vi "Read Configuration Parameters.vi"(8 "error in (no error)":errorcluster, 10 "refnum":T1, 11 "Configuration in":refnum<class "Configuration.lvclass">) -> (0 "error out":errorcluster, 2 "refnum out":T1, 3 "Configuration out":refnum<class "Configuration.lvclass">)   [LabVIEW 2016, in "Configuration.lvlib" / "Configuration.lvclass"]
uses:
  <userlib>/Configuration Dialog Actor/Configuration.lvclass
  <vilib>/Utility/config.llb/Config Data RefNum.ctl
  <userlib>/Configuration Dialog Actor/Configuration.lvclass/Configuration.ctl
  <vilib>/Utility/config.llb/NI_LVConfig.lvlib
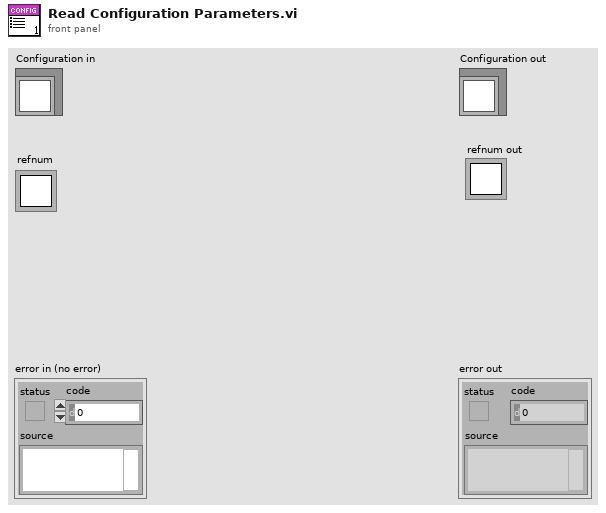
[diagram p1: front panel]
types:
  T1 = typedef "NI_LVConfig.lvlib/Config Data RefNum.ctl" = refnum<k1>
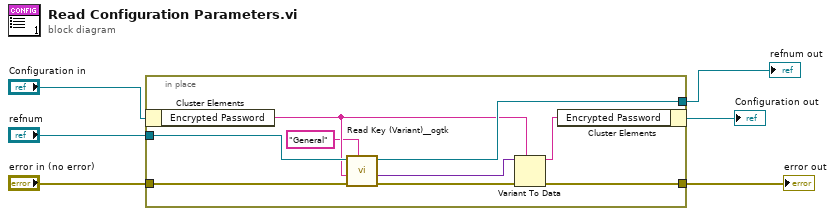
[diagram p0: block diagram]
diagram:
  n1 = in-place {
    in-place-border: "refnum" -> [w15]
    in-place-border: [w14] -> w5
    in-place-border: "error in (no error)" -> [w13]
    in-place-border: [w10] -> w3
    n2 = in-place-cluster #1("Configuration in") -> ("Encrypted Password"=w12:string)
    n3 = call <userlib>:"Read Key (Variant)__ogtk.vi"("section"="General", "error in (no error)"=w13, "type"=w12, "refnum"=w15) -> ("error out"=w11:errorcluster, "key-value"=w7:variant, "refnum out"=w14:T1)  [unwired: 4 in, 1 out]
    n4 = Variant To Data(error in=w11, type=w12, Variant=w7) -> (data=w8:string, error out=w10:errorcluster)
    n5 = in-place-cluster #1("Encrypted Password"=w8) -> (→"Configuration out":refnum<class "Configuration.lvclass">)
  }
  "error out" <- w3
  "refnum out" <- w5
